vi "Test_ReverseInsertItems.vi"(8 "error in (no error)":errorcluster, 11 "TestCase in":refnum<class "ListImp_Functional.lvclass">) -> (0 "error out":errorcluster, 3 "TestCase out":refnum<class "ListImp_Functional.lvclass">)   [LabVIEW 2009, in "ListImp_Functional.lvclass"]
uses:
  ListImp_Functional.lvclass
  ListImp_Functional.lvclass/ListImp_Functional.ctl
  source/Lists/List/List.lvclass
  source/Lists.Interfaces/String/String.lvclass
  UnitTestComparisons/UnitTestComparisons.lvlib
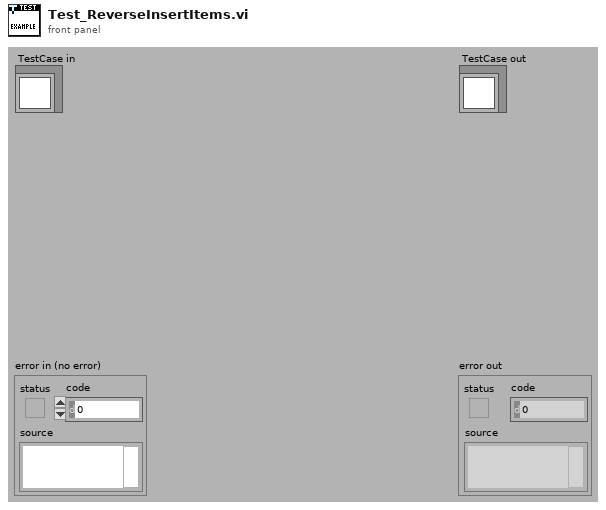
[diagram p1: front panel]
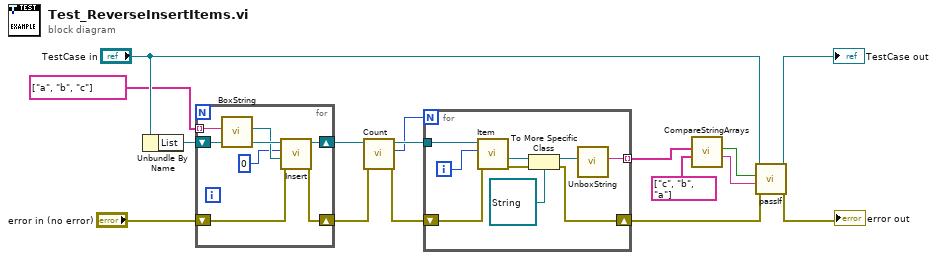
[diagram p0: block diagram]
diagram:
  n1 = Unbundle By Name("TestCase in") -> ("List"=w13:refnum<class "List.lvclass">)
  n2 = for {
    tunnel: string[] ["a", "b", "c"] -> [w20] mode=indexing
    shift-right: [w22] -> w9
    shift-left: w13 -> [w23]
    shift-right: [w18] -> w6
    shift-left: "error in (no error)" -> [w19]
    n3 = call "BoxString.vi"("String"=w20) -> ("String out"=w21:refnum<class "String.lvclass">)  [unwired: 10 in]
    n4 = call-dynamic "Insert.vi"("error in (no error)"=w19, "Item"=w21, "Index"=0, "List in"=w23) -> ("error out"=w18:errorcluster, "List out"=w22:refnum<class "List.lvclass">)  [unwired: 6 in]
  }
  n5 = call-dynamic "Count.vi"("error in (no error)"=w6, "List in"=w9) -> ("error out"=w5:errorcluster, "Number of Items"=w7:i32, "List out"=w8:refnum<class "List.lvclass">)  [unwired: 7 in]
  n6 = for {
    N: w7 -> [_]
    tunnel: w8 -> [w32]
    shift-right: [w26] -> w11
    shift-left: w5 -> [w31]
    tunnel: [w24] -> w4 mode=indexing
    i -> [w30]
    n7 = call-dynamic "Item.vi"("error in (no error)"=w31, "Index"=w30, "List in"=w32) -> ("error out"=w27:errorcluster, "Item"=w29:refnum<class>)  [unwired: 6 in, 1 out]
    n8 = To More Specific Class(target class=refnum<class "String.lvclass"> refnum ("LapDog.Collections.v0.Lists.Interfaces.lvlib:String.lvclass"), reference=w29, error in=w27) -> (specific class reference=w28:refnum<class "String.lvclass">, error out=w26:errorcluster)
    n9 = call "UnboxString.vi"("String in"=w28) -> ("String"=w24:string)  [unwired: 10 in]
  }
  n10 = call "CompareStringArrays.vi"("Expected Strings"=string[] ["c", "b", "a"], "Actual Strings"=w4) -> ("Message"=w1:string, "Equal?"=w2:bool)  [unwired: 8 in]
  n11 = call-dynamic "passIf.vi"("error in (no error)"=w11, "message (\"\")"=w1, "pass"=w2, "TestCase in"="TestCase in") -> ("error out"=→"error out":errorcluster, "TestCase out"=→"TestCase out":refnum<class "ListImp_Functional.lvclass">)  [unwired: 6 in]
